vi "Road Accident Detection and Alert System.vi"() -> ()   [LabVIEW 2020]
panel:
  out "Boolean":bool
  out "Z":dbl(graph)
  out "Y":dbl(graph)
  out "X":dbl(graph)
  in  "VISA resource name":refnum<visa-resource-name>
  in  "Emergency Table Control":string[][](table)
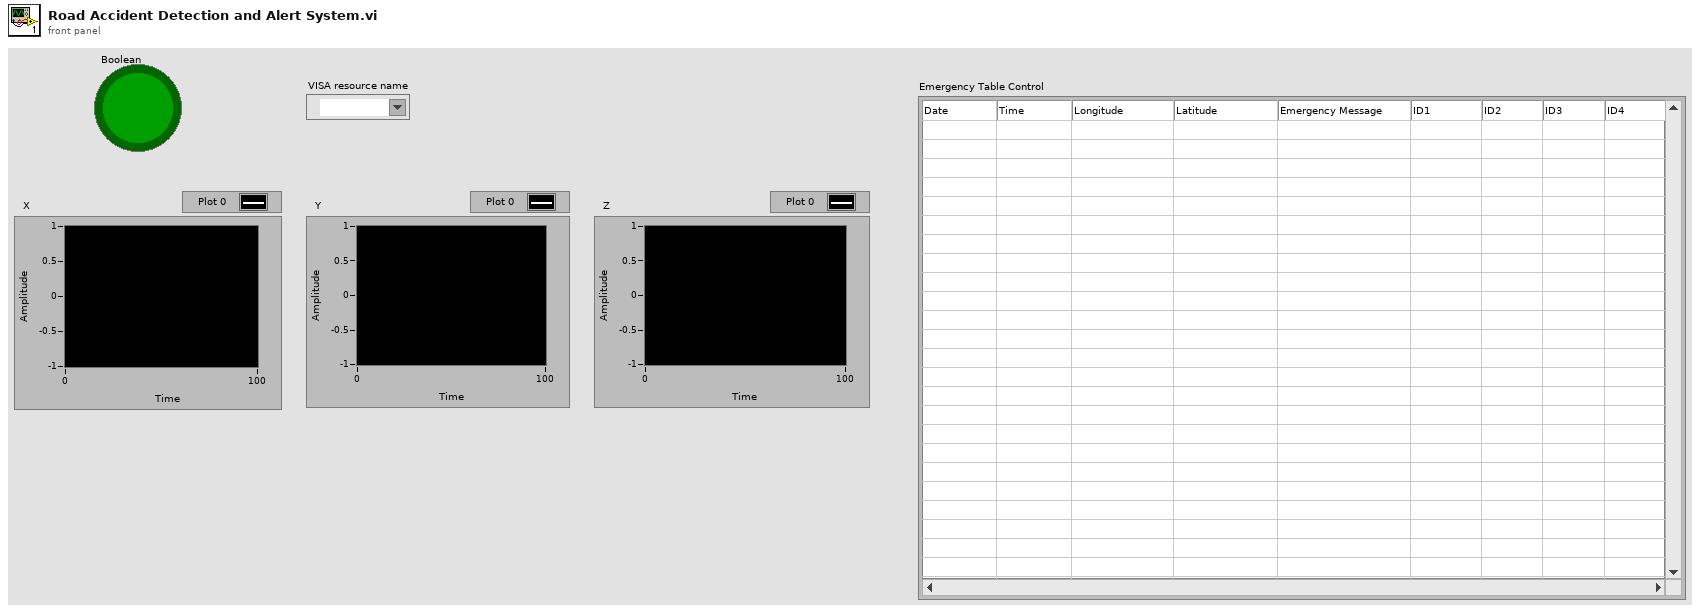
[diagram p1: front panel]
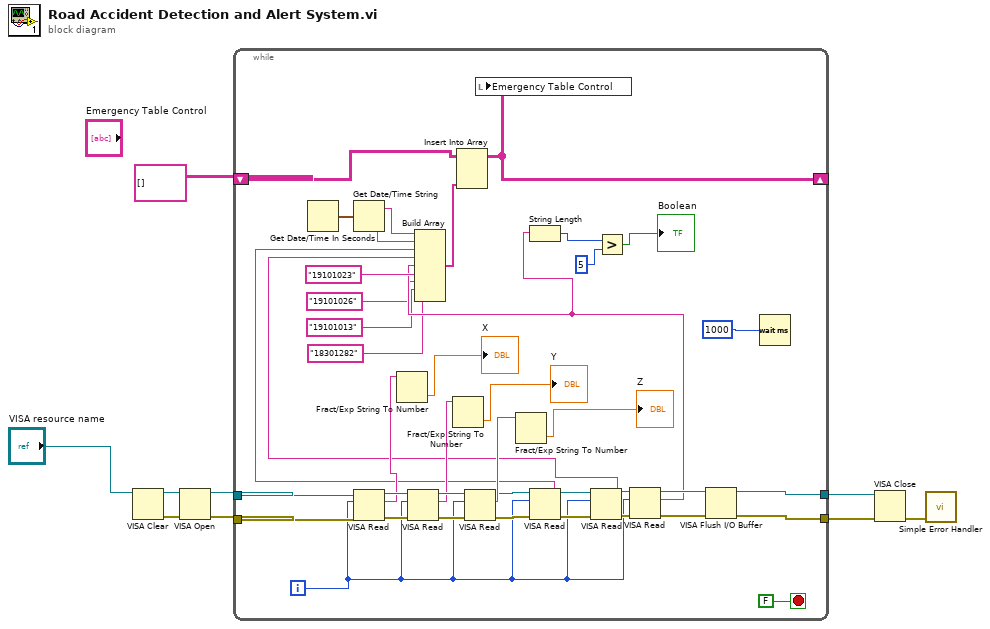
[diagram p0: block diagram]
diagram:
  n1 = VISA Clear(VISA resource name="VISA resource name") -> (VISA resource name out=w8:refnum<visa-resource-name>, error out=w9:errorcluster)  [unwired: 1 in]
  n2 = VISA Open(error in (no error)=w9, VISA resource name=w8) -> (VISA resource name=w7:refnum<visa-resource-name>, error out=w6:errorcluster)  [unwired: 3 in]
  n3 = while {
    tunnel: w7 -> [w35]
    tunnel: w6 -> [w34]
    shift-right: [w48] -> _
    shift-left: string[][] [] -> [w49]
    tunnel: [w42] -> w3
    tunnel: [w41] -> w1
    i -> [w18]
    stop <- FALSE stop-if-true
    n4 = Get Date/Time In Seconds() -> (seconds since 1Jan1904=w47:timestamp)
    n5 = Get Date/Time String(seconds (now)=w47) -> (date string=w46:string, time string=w45:string)  [unwired: 2 in]
    n6 = VISA Read(VISA resource name=w35, byte count=w18, error in (no error)=w34) -> (VISA resource name out=w39:refnum<visa-resource-name>, read buffer=w33:string, error out=w38:errorcluster)  [unwired: 1 out]
    n7 = Fract/Exp String To Number(string=w33) -> (number=→"X":dbl)  [unwired: 3 in, 1 out]
    n8 = VISA Read(VISA resource name=w39, byte count=w18, error in (no error)=w38) -> (VISA resource name out=w37:refnum<visa-resource-name>, read buffer=w32:string, error out=w36:errorcluster)  [unwired: 1 out]
    n9 = Fract/Exp String To Number(string=w32) -> (number=→"Y":dbl)  [unwired: 3 in, 1 out]
    n10 = VISA Read(VISA resource name=w37, byte count=w18, error in (no error)=w36) -> (VISA resource name out=w23:refnum<visa-resource-name>, read buffer=w28:string, error out=w22:errorcluster)  [unwired: 1 out]
    n11 = Fract/Exp String To Number(string=w28) -> (number=→"Z":dbl)  [unwired: 3 in, 1 out]
    n12 = VISA Read(VISA resource name=w23, byte count=w18, error in (no error)=w22) -> (VISA resource name out=w21:refnum<visa-resource-name>, read buffer=w19:string, error out=w20:errorcluster)  [unwired: 1 out]
    n13 = VISA Read(VISA resource name=w21, byte count=w18, error in (no error)=w20) -> (VISA resource name out=w27:refnum<visa-resource-name>, read buffer=w17:string, error out=w24:errorcluster)  [unwired: 1 out]
    n14 = VISA Read(VISA resource name=w27, byte count=w18, error in (no error)=w24) -> (VISA resource name out=w26:refnum<visa-resource-name>, read buffer=w16:string, error out=w25:errorcluster)  [unwired: 1 out]
    n15 = Build Array(w46, w45, w19, w17, w16, "19101023" ("element"), "19101026" ("element"), "19101013" ("element"), "18301282" ("element")) -> (w44:string[])
    n16 = Insert Into Array(array=w49, new element=w44) -> (w48:string[][])  [unwired: 2 in]
    n17 = local write "Emergency Table Control"(w48) -> ()
    n18 = String Length(string=w16) -> (length=w15:i32)
    n19 = Greater?(x=w15, y=5) -> (0:→"Boolean":bool)
    n20 = VISA Flush I/O Buffer(VISA resource name=w26, error in (no error)=w25) -> (VISA resource name out=w42:refnum<visa-resource-name>, error out=w41:errorcluster)  [unwired: 1 in]
    n21 = Wait (ms)(milliseconds to wait=u32 1000) -> ()  [unwired: 1 out]
  }
  n22 = VISA Close(VISA resource name=w3, error in (no error)=w1) -> (error out=w2:errorcluster)
  n23 = call <vilib>:"Simple Error Handler.vi"("error in (no error)"=w2) -> ()  [unwired: 4 in, 5 out]
